vi "tsdb_get_flexray_frame_properties_by_index_verbose.vi"(8 "error in (no error)":errorcluster caption="错误输入（无错误）", 10 "ADBIndex":i32, 11 "path in":path) -> (0 "error out":errorcluster caption="错误输出", 1 "flexray_frame_properties_by_index":T1, 2 "function return":i32, 3 "path out":path)   [LabVIEW 2014]
doc: "Function introduction: Retrieve flexray frame attribute information through indexing\nCall location\nInput parameter ADB Index: database index\nAECUIndes: ECU index\nAFrameIndex：\n Frame index\nAIsTx：\n TX AFRChannelMask: Channel Mask\nAFRBaseCycle：\n Basic cycle\nAFRCycleRepetition：\n Repetitive cycle\nAFRIsStartupFrame：\n Is it the starting frame\nAFRSlotId：slotId AFRCycleMask：\n Periodic mask\nASignalCount：\n Number of signals\nAFRDLC: DLC length\nAName：\n Database Name\nAComment：\n notes\nReturn value 0: Successful execution\nOther values: Failed"
uses:
  Typedef/FlexRay/flexray_frame_properties_by_index.ctl
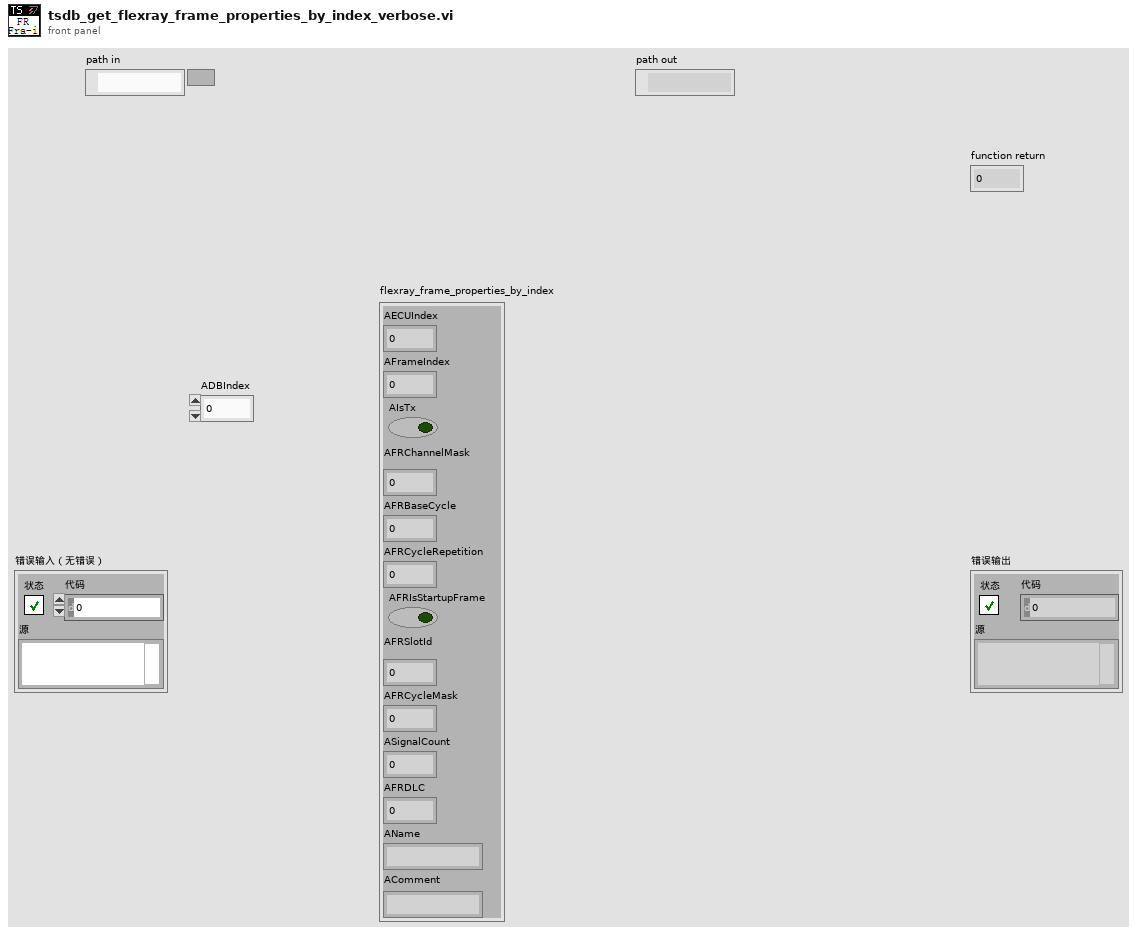
[diagram p1: front panel]
types:
  T1 = typedef "flexray_frame_properties_by_index.ctl" = cluster{"AECUIndex":i32, "AFrameIndex":i32, "AIsTx":bool, "AFRChannelMask":i32, "AFRBaseCycle":i32, "AFRCycleRepetition":i32, "AFRIsStartupFrame":bool, "AFRSlotId":i32, "AFRCycleMask":i64, "ASignalCount":i32, "AFRDLC":i32, "AName":string, "AComment":string}
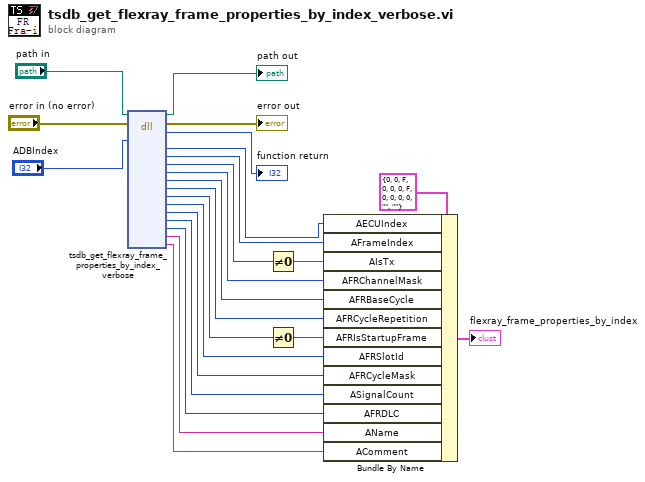
[diagram p0: block diagram]
diagram:
  n1 = dll-call lib="D:/Work/LabVIEW Code/TSMaster Labview SDK/LabVIEW/LabVIEW-TSMasterAPI_CLN/TSMasterAPI_LabVIEW-2024-10-08 14-20-13/Not_organized_vi/TSMaster.*" fn="tsdb_get_flexray_frame_properties_by_index_verbose"(path in="path in", error in="error in (no error)", "ADBIndex"="ADBIndex") -> (path out=→"path out":path, error out=→"error out":errorcluster, "返回类型"=→"function return":i32, "AECUIndex"=w14:i32, "AFrameIndex"=w13:i32, "AIsTx"=w2:u8, "AFRChannelMask"=w12:i32, "AFRBaseCycle"=w11:i32, "AFRCycleRepetition"=w10:i32, "AFRIsStartupFrame"=w22:u8, "AFRSlotId"=w9:i32, "AFRCycleMask"=w8:i64, "ASignalCount"=w7:i32, "AFRDLC"=w6:i32, "AName"=w5:string, "AComment"=w4:string)  [unwired: 15 in]
  n2 = Not Equal To 0?(x=w2) -> (x != 0?=w1:bool)
  n3 = Not Equal To 0?(x=w22) -> (x != 0?=w3:bool)
  n4 = Bundle By Name(cluster=T1 {"AECUIndex"=0, "AFrameIndex"=0, "AIsTx"=FALSE, "AFRChannelMask"=0, "AFRBaseCycle"=0, "AFRCycleRepetition"=0, "AFRIsStartupFrame"=FALSE, "AFRSlotId"=0, "AFRCycleMask"=0, "ASignalCount"=0, "AFRDLC"=0, "AName"="", "AComment"=""} ("flexray_frame_properties_by_index"), "AECUIndex"=w14, "AFrameIndex"=w13, "AIsTx"=w1, "AFRChannelMask"=w12, "AFRBaseCycle"=w11, "AFRCycleRepetition"=w10, "AFRIsStartupFrame"=w3, "AFRSlotId"=w9, "AFRCycleMask"=w8, "ASignalCount"=w7, "AFRDLC"=w6, "AName"=w5, "AComment"=w4) -> (→"flexray_frame_properties_by_index":T1)
